vi "Experiment 26.vi"() -> ()   [LabVIEW 2026]
doc: "Experiment 26\nThis experiment (26) is like experiment 25 but uses 11 loops instead of 10. The subVIs in the first five loops use \"Same as caller\", and the last 6 loops use \"Other 1\"."
uses:
  <vilib>/AdvancedString/1D String Array to Delimited String (string).vi
  <vilib>/Analysis/baseanly.llb/Mean (DBL).vi
  <vilib>/Analysis/NI_AALBase.lvlib
panel:
  out "No. Of Iterations Executed - Loop 11":i32
  out "Output - Loop 11":dbl[](array[numeric]) format="%.3f"
  out "No. Of Iterations As Block Of Text (easy to copy into Excel)":string
  out "No. Of Iterations Executed - Loop 10":i32
  out "Output - Loop 10":dbl[](array[numeric]) format="%.3f"
  out "No. Of Iterations Executed - Loop 9":i32
  out "Output - Loop 9":dbl[](array[numeric]) format="%.3f"
  out "No. Of Iterations Executed - Loop 8":i32
  out "Output - Loop 8":dbl[](array[numeric]) format="%.3f"
  out "No. Of Iterations Executed - Loop 7":i32
  out "Output - Loop 7":dbl[](array[numeric]) format="%.3f"
  out "No. Of Iterations Executed - Loop 6":i32
  out "Output - Loop 6":dbl[](array[numeric]) format="%.3f"
  out "No. Of Iterations Executed - Loop 5":i32
  out "Output - Loop 5":dbl[](array[numeric]) format="%.3f"
  out "No. Of Iterations Executed - Loop 4":i32
  out "Output - Loop 4":dbl[](array[numeric]) format="%.3f"
  out "No. Of Iterations Executed - Loop 3":i32
  out "Output - Loop 3":dbl[](array[numeric]) format="%.3f"
  out "Avg. No. Of Iterations Executed - All Loops":dbl format="%.1f"
  out "No. Of Iterations Executed - Loop 2":i32
  out "Output - Loop 2":dbl[](array[numeric]) format="%.3f"
  out "No. Of Iterations Executed - Loop 1":i32
  out "Output - Loop 1":dbl[](array[numeric]) format="%.3f"
  out "Stop VI?":bool
  # "Experiment 26"
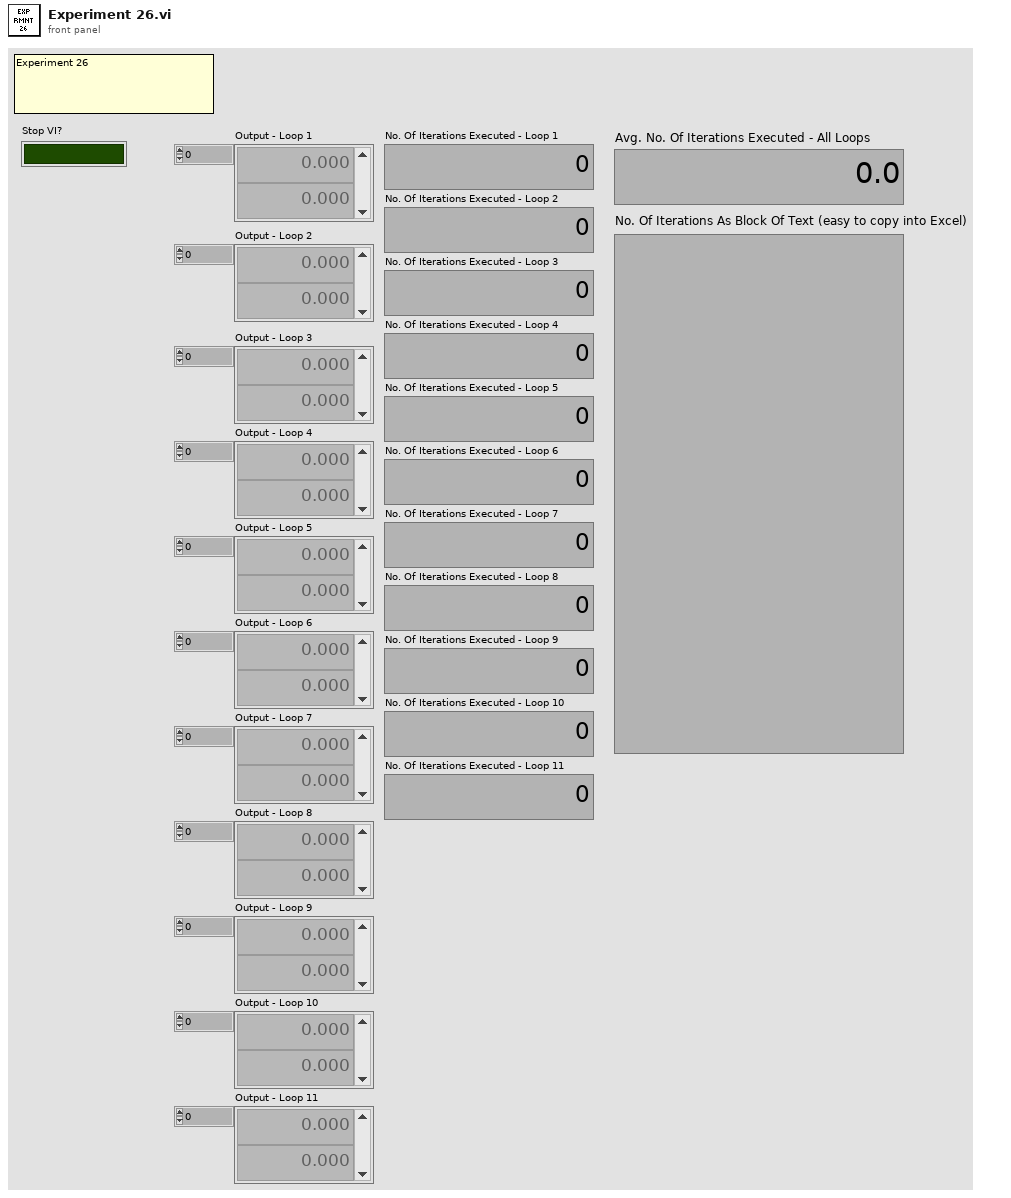
[diagram p1: front panel]
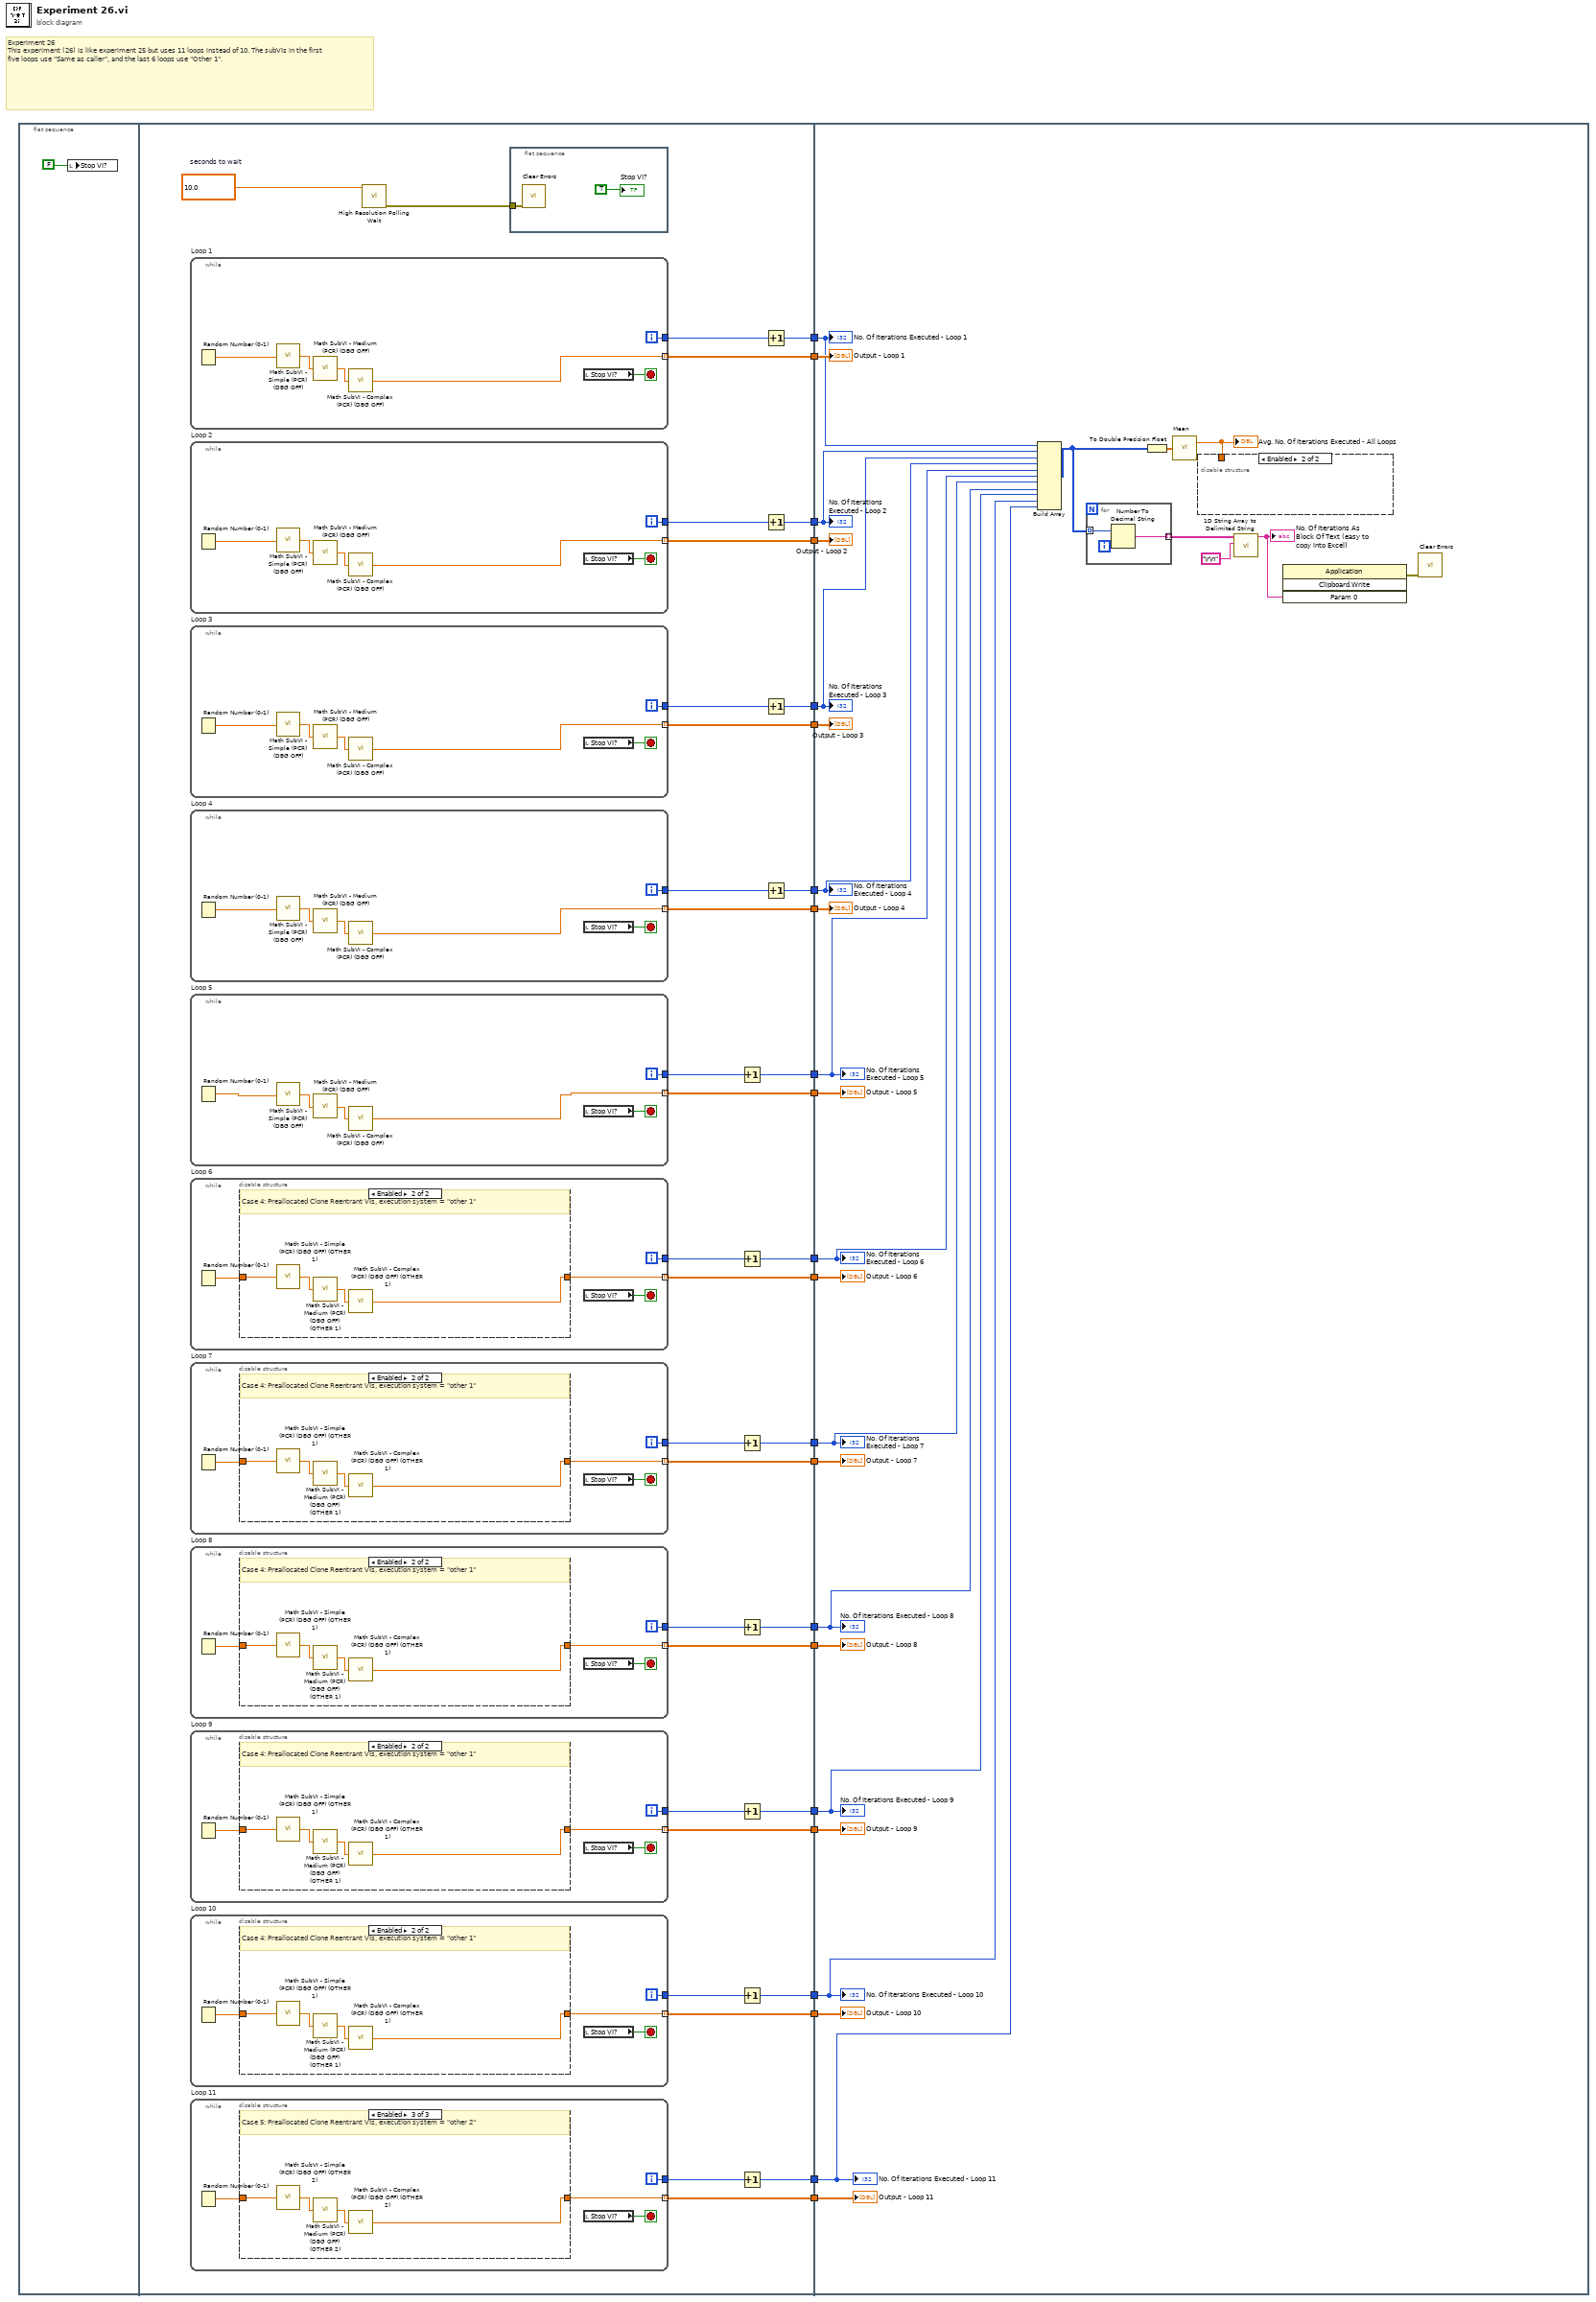
[diagram p0: block diagram]
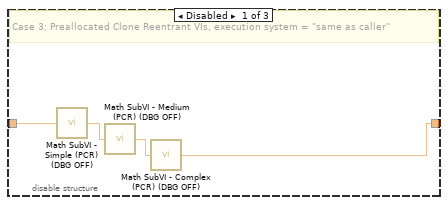
[diagram p2: hidden frame]
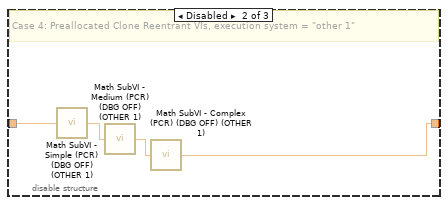
[diagram p3: hidden frame]
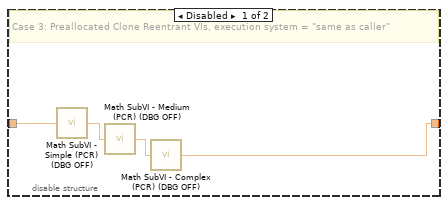
[diagram p4: hidden frame]
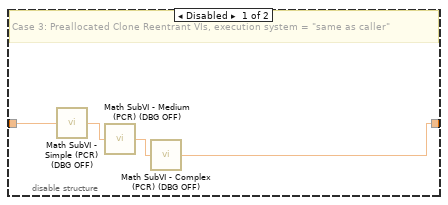
[diagram p5: hidden frame]
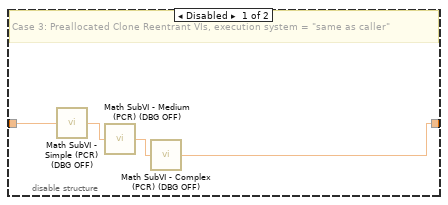
[diagram p6: hidden frame]
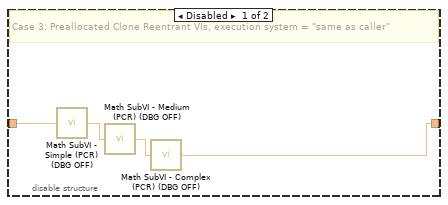
[diagram p7: hidden frame]
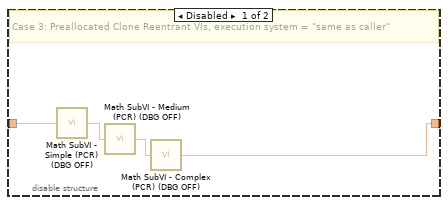
[diagram p8: hidden frame]
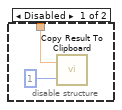
[diagram p9: hidden frame]
diagram:
  # "Experiment 26\nThis experiment (26) is like experiment 25 but uses 11 loops instead of 10. The subVIs in the first five loops use \"Same as caller\", and the last 6 loops use \"Other 1\"."
  n1 = flat-sequence {
    tunnel: [w56] -> w22
    tunnel: [w54] -> w21
    tunnel: [w53] -> w20
    tunnel: [w44] -> w19
    tunnel: [w52] -> w18
    tunnel: [w42] -> w17
    tunnel: [w40] -> w16
    tunnel: [w51] -> w15
    tunnel: [w38] -> w14
    tunnel: [w50] -> w13
    tunnel: [w36] -> w12
    tunnel: [w45] -> w11
    tunnel: [w34] -> w10
    tunnel: [w46] -> w9
    tunnel: [w32] -> w8
    tunnel: [w47] -> w7
    tunnel: [w30] -> w6
    tunnel: [w48] -> w5
    tunnel: [w27] -> w4
    tunnel: [w49] -> w3
    tunnel: [w26] -> w2
    tunnel: [w24] -> w1
    tunnel: w22 -> [w195]
    tunnel: w21 -> [w193]
    tunnel: w20 -> [w192]
    tunnel: w19 -> [w194]
    tunnel: w18 -> [w188]
    tunnel: w17 -> [w190]
    tunnel: w16 -> [w189]
    tunnel: w15 -> [w187]
    tunnel: w14 -> [w185]
    tunnel: w13 -> [w179]
    tunnel: w12 -> [w184]
    tunnel: w11 -> [w178]
    tunnel: w10 -> [w183]
    tunnel: w9 -> [w177]
    tunnel: w8 -> [w182]
    tunnel: w7 -> [w176]
    tunnel: w6 -> [w181]
    tunnel: w5 -> [w175]
    tunnel: w4 -> [w180]
    tunnel: w3 -> [w174]
    tunnel: w2 -> [w168]
    tunnel: w1 -> [w167]
    frame #0 {
      n2 = local write "Stop VI?"(FALSE) -> ()
    }
    frame #1 {
      w58 = 10.0  # seconds to wait
      n3 = while "Loop 1" {
        tunnel: [w162] -> w56 mode=indexing
        tunnel: [w163] -> w55
        i -> [w163]
        stop <- w164 stop-if-true
        n4 = Random Number (0-1)() -> (number: 0 to 1=w161:dbl)
        n5 = call "Math SubVI - Simple (PCR) (DBG OFF).vi"("Input"=w161) -> ("Output"=w159:dbl)
        n6 = call "Math SubVI - Medium (PCR) (DBG OFF).vi"("Input"=w159) -> ("Output"=w160:dbl)
        n7 = call "Math SubVI - Complex (PCR) (DBG OFF).vi"("Input"=w160) -> ("Output"=w162:dbl)
        n8 = local read "Stop VI?"() -> (w164:bool)
      }
      n9 = while "Loop 2" {
        tunnel: [w155] -> w44 mode=indexing
        tunnel: [w157] -> w43
        i -> [w157]
        stop <- w158 stop-if-true
        n10 = Random Number (0-1)() -> (number: 0 to 1=w156:dbl)
        n11 = call "Math SubVI - Simple (PCR) (DBG OFF).vi"("Input"=w156) -> ("Output"=w153:dbl)
        n12 = call "Math SubVI - Medium (PCR) (DBG OFF).vi"("Input"=w153) -> ("Output"=w154:dbl)
        n13 = call "Math SubVI - Complex (PCR) (DBG OFF).vi"("Input"=w154) -> ("Output"=w155:dbl)
        n14 = local read "Stop VI?"() -> (w158:bool)
      }
      n15 = while "Loop 3" {
        tunnel: [w149] -> w42 mode=indexing
        tunnel: [w151] -> w41
        i -> [w151]
        stop <- w152 stop-if-true
        n16 = Random Number (0-1)() -> (number: 0 to 1=w150:dbl)
        n17 = call "Math SubVI - Simple (PCR) (DBG OFF).vi"("Input"=w150) -> ("Output"=w147:dbl)
        n18 = call "Math SubVI - Medium (PCR) (DBG OFF).vi"("Input"=w147) -> ("Output"=w148:dbl)
        n19 = call "Math SubVI - Complex (PCR) (DBG OFF).vi"("Input"=w148) -> ("Output"=w149:dbl)
        n20 = local read "Stop VI?"() -> (w152:bool)
      }
      n21 = while "Loop 4" {
        tunnel: [w143] -> w40 mode=indexing
        tunnel: [w145] -> w39
        i -> [w145]
        stop <- w146 stop-if-true
        n22 = Random Number (0-1)() -> (number: 0 to 1=w144:dbl)
        n23 = call "Math SubVI - Simple (PCR) (DBG OFF).vi"("Input"=w144) -> ("Output"=w141:dbl)
        n24 = call "Math SubVI - Medium (PCR) (DBG OFF).vi"("Input"=w141) -> ("Output"=w142:dbl)
        n25 = call "Math SubVI - Complex (PCR) (DBG OFF).vi"("Input"=w142) -> ("Output"=w143:dbl)
        n26 = local read "Stop VI?"() -> (w146:bool)
      }
      n27 = while "Loop 5" {
        tunnel: [w137] -> w38 mode=indexing
        tunnel: [w139] -> w37
        i -> [w139]
        stop <- w140 stop-if-true
        n28 = Random Number (0-1)() -> (number: 0 to 1=w138:dbl)
        n29 = call "Math SubVI - Simple (PCR) (DBG OFF).vi"("Input"=w138) -> ("Output"=w135:dbl)
        n30 = call "Math SubVI - Medium (PCR) (DBG OFF).vi"("Input"=w135) -> ("Output"=w136:dbl)
        n31 = call "Math SubVI - Complex (PCR) (DBG OFF).vi"("Input"=w136) -> ("Output"=w137:dbl)
        n32 = local read "Stop VI?"() -> (w140:bool)
      }
      n33 = while "Loop 6" {
        tunnel: [w123] -> w36 mode=indexing
        tunnel: [w125] -> w35
        i -> [w125]
        stop <- w126 stop-if-true
        n34 = Random Number (0-1)() -> (number: 0 to 1=w124:dbl)
        n35 = disable-structure shown="Enabled" {
          disable-tunnel: w124 -> [w130 w134]
          disable-tunnel: [w129 w133] -> w123
          frame Disabled {
            # "Case 3: Preallocated Clone Reentrant VIs, execution system = \"same as caller\""
            n36 = call "Math SubVI - Simple (PCR) (DBG OFF).vi"("Input"=w130) -> ("Output"=w127:dbl)
            n37 = call "Math SubVI - Medium (PCR) (DBG OFF).vi"("Input"=w127) -> ("Output"=w128:dbl)
            n38 = call "Math SubVI - Complex (PCR) (DBG OFF).vi"("Input"=w128) -> ("Output"=w129:dbl)
          }
          frame Enabled {
            # "Case 4: Preallocated Clone Reentrant VIs, execution system = \"other 1\""
            n39 = call "Math SubVI - Simple (PCR) (DBG OFF) (OTHER 1).vi"("Input"=w134) -> ("Output"=w131:dbl)
            n40 = call "Math SubVI - Medium (PCR) (DBG OFF) (OTHER 1).vi"("Input"=w131) -> ("Output"=w132:dbl)
            n41 = call "Math SubVI - Complex (PCR) (DBG OFF) (OTHER 1).vi"("Input"=w132) -> ("Output"=w133:dbl)
          }
        }
        n42 = local read "Stop VI?"() -> (w126:bool)
      }
      n43 = while "Loop 7" {
        tunnel: [w111] -> w34 mode=indexing
        tunnel: [w113] -> w33
        i -> [w113]
        stop <- w114 stop-if-true
        n44 = Random Number (0-1)() -> (number: 0 to 1=w112:dbl)
        n45 = disable-structure shown="Enabled" {
          disable-tunnel: w112 -> [w118 w122]
          disable-tunnel: [w117 w121] -> w111
          frame Disabled {
            # "Case 3: Preallocated Clone Reentrant VIs, execution system = \"same as caller\""
            n46 = call "Math SubVI - Simple (PCR) (DBG OFF).vi"("Input"=w118) -> ("Output"=w115:dbl)
            n47 = call "Math SubVI - Medium (PCR) (DBG OFF).vi"("Input"=w115) -> ("Output"=w116:dbl)
            n48 = call "Math SubVI - Complex (PCR) (DBG OFF).vi"("Input"=w116) -> ("Output"=w117:dbl)
          }
          frame Enabled {
            # "Case 4: Preallocated Clone Reentrant VIs, execution system = \"other 1\""
            n49 = call "Math SubVI - Simple (PCR) (DBG OFF) (OTHER 1).vi"("Input"=w122) -> ("Output"=w119:dbl)
            n50 = call "Math SubVI - Medium (PCR) (DBG OFF) (OTHER 1).vi"("Input"=w119) -> ("Output"=w120:dbl)
            n51 = call "Math SubVI - Complex (PCR) (DBG OFF) (OTHER 1).vi"("Input"=w120) -> ("Output"=w121:dbl)
          }
        }
        n52 = local read "Stop VI?"() -> (w114:bool)
      }
      n53 = while "Loop 8" {
        tunnel: [w99] -> w32 mode=indexing
        tunnel: [w101] -> w31
        i -> [w101]
        stop <- w102 stop-if-true
        n54 = Random Number (0-1)() -> (number: 0 to 1=w100:dbl)
        n55 = disable-structure shown="Enabled" {
          disable-tunnel: w100 -> [w106 w110]
          disable-tunnel: [w105 w109] -> w99
          frame Disabled {
            # "Case 3: Preallocated Clone Reentrant VIs, execution system = \"same as caller\""
            n56 = call "Math SubVI - Simple (PCR) (DBG OFF).vi"("Input"=w106) -> ("Output"=w103:dbl)
            n57 = call "Math SubVI - Medium (PCR) (DBG OFF).vi"("Input"=w103) -> ("Output"=w104:dbl)
            n58 = call "Math SubVI - Complex (PCR) (DBG OFF).vi"("Input"=w104) -> ("Output"=w105:dbl)
          }
          frame Enabled {
            # "Case 4: Preallocated Clone Reentrant VIs, execution system = \"other 1\""
            n59 = call "Math SubVI - Simple (PCR) (DBG OFF) (OTHER 1).vi"("Input"=w110) -> ("Output"=w107:dbl)
            n60 = call "Math SubVI - Medium (PCR) (DBG OFF) (OTHER 1).vi"("Input"=w107) -> ("Output"=w108:dbl)
            n61 = call "Math SubVI - Complex (PCR) (DBG OFF) (OTHER 1).vi"("Input"=w108) -> ("Output"=w109:dbl)
          }
        }
        n62 = local read "Stop VI?"() -> (w102:bool)
      }
      n63 = while "Loop 9" {
        tunnel: [w87] -> w30 mode=indexing
        tunnel: [w89] -> w29
        i -> [w89]
        stop <- w90 stop-if-true
        n64 = Random Number (0-1)() -> (number: 0 to 1=w88:dbl)
        n65 = disable-structure shown="Enabled" {
          disable-tunnel: w88 -> [w94 w98]
          disable-tunnel: [w93 w97] -> w87
          frame Disabled {
            # "Case 3: Preallocated Clone Reentrant VIs, execution system = \"same as caller\""
            n66 = call "Math SubVI - Simple (PCR) (DBG OFF).vi"("Input"=w94) -> ("Output"=w91:dbl)
            n67 = call "Math SubVI - Medium (PCR) (DBG OFF).vi"("Input"=w91) -> ("Output"=w92:dbl)
            n68 = call "Math SubVI - Complex (PCR) (DBG OFF).vi"("Input"=w92) -> ("Output"=w93:dbl)
          }
          frame Enabled {
            # "Case 4: Preallocated Clone Reentrant VIs, execution system = \"other 1\""
            n69 = call "Math SubVI - Simple (PCR) (DBG OFF) (OTHER 1).vi"("Input"=w98) -> ("Output"=w95:dbl)
            n70 = call "Math SubVI - Medium (PCR) (DBG OFF) (OTHER 1).vi"("Input"=w95) -> ("Output"=w96:dbl)
            n71 = call "Math SubVI - Complex (PCR) (DBG OFF) (OTHER 1).vi"("Input"=w96) -> ("Output"=w97:dbl)
          }
        }
        n72 = local read "Stop VI?"() -> (w90:bool)
      }
      n73 = while "Loop 10" {
        tunnel: [w75] -> w27 mode=indexing
        tunnel: [w77] -> w28
        i -> [w77]
        stop <- w78 stop-if-true
        n74 = Random Number (0-1)() -> (number: 0 to 1=w76:dbl)
        n75 = disable-structure shown="Enabled" {
          disable-tunnel: w76 -> [w82 w86]
          disable-tunnel: [w81 w85] -> w75
          frame Disabled {
            # "Case 3: Preallocated Clone Reentrant VIs, execution system = \"same as caller\""
            n76 = call "Math SubVI - Simple (PCR) (DBG OFF).vi"("Input"=w82) -> ("Output"=w79:dbl)
            n77 = call "Math SubVI - Medium (PCR) (DBG OFF).vi"("Input"=w79) -> ("Output"=w80:dbl)
            n78 = call "Math SubVI - Complex (PCR) (DBG OFF).vi"("Input"=w80) -> ("Output"=w81:dbl)
          }
          frame Enabled {
            # "Case 4: Preallocated Clone Reentrant VIs, execution system = \"other 1\""
            n79 = call "Math SubVI - Simple (PCR) (DBG OFF) (OTHER 1).vi"("Input"=w86) -> ("Output"=w83:dbl)
            n80 = call "Math SubVI - Medium (PCR) (DBG OFF) (OTHER 1).vi"("Input"=w83) -> ("Output"=w84:dbl)
            n81 = call "Math SubVI - Complex (PCR) (DBG OFF) (OTHER 1).vi"("Input"=w84) -> ("Output"=w85:dbl)
          }
        }
        n82 = local read "Stop VI?"() -> (w78:bool)
      }
      n83 = while "Loop 11" {
        tunnel: [w59] -> w26 mode=indexing
        tunnel: [w61] -> w25
        i -> [w61]
        stop <- w62 stop-if-true
        n84 = Random Number (0-1)() -> (number: 0 to 1=w60:dbl)
        n85 = disable-structure shown="Enabled" {
          disable-tunnel: w60 -> [w66 w70 w74]
          disable-tunnel: [w65 w69 w73] -> w59
          frame Disabled {
            # "Case 3: Preallocated Clone Reentrant VIs, execution system = \"same as caller\""
            n86 = call "Math SubVI - Simple (PCR) (DBG OFF).vi"("Input"=w66) -> ("Output"=w63:dbl)
            n87 = call "Math SubVI - Medium (PCR) (DBG OFF).vi"("Input"=w63) -> ("Output"=w64:dbl)
            n88 = call "Math SubVI - Complex (PCR) (DBG OFF).vi"("Input"=w64) -> ("Output"=w65:dbl)
          }
          frame Disabled {
            # "Case 4: Preallocated Clone Reentrant VIs, execution system = \"other 1\""
            n89 = call "Math SubVI - Simple (PCR) (DBG OFF) (OTHER 1).vi"("Input"=w70) -> ("Output"=w67:dbl)
            n90 = call "Math SubVI - Medium (PCR) (DBG OFF) (OTHER 1).vi"("Input"=w67) -> ("Output"=w68:dbl)
            n91 = call "Math SubVI - Complex (PCR) (DBG OFF) (OTHER 1).vi"("Input"=w68) -> ("Output"=w69:dbl)
          }
          frame Enabled {
            # "Case 5: Preallocated Clone Reentrant VIs, execution system = \"other 2\""
            n92 = call "Math SubVI - Simple (PCR) (DBG OFF) (OTHER 2).vi"("Input"=w74) -> ("Output"=w71:dbl)
            n93 = call "Math SubVI - Medium (PCR) (DBG OFF) (OTHER 2).vi"("Input"=w71) -> ("Output"=w72:dbl)
            n94 = call "Math SubVI - Complex (PCR) (DBG OFF) (OTHER 2).vi"("Input"=w72) -> ("Output"=w73:dbl)
          }
        }
        n95 = local read "Stop VI?"() -> (w62:bool)
      }
      n96 = call <vilib>:"High Resolution Polling Wait.vi"("seconds to wait"=w58) -> ("error out"=w57:errorcluster)  [unwired: 10 in]
      n97 = flat-sequence {
        tunnel: w57 -> [w165]
        frame #0 {
          n98 = call <vilib>:"Clear Errors.vi"("error in (no error)"=w165) -> ()  [unwired: 5 in, 2 out]
          "Stop VI?" <- TRUE
        }
      }
      n99 = Increment(x=w37) -> (x+1=w50:i32)
      n100 = Increment(x=w35) -> (x+1=w45:i32)
      n101 = Increment(x=w33) -> (x+1=w46:i32)
      n102 = Increment(x=w31) -> (x+1=w47:i32)
      n103 = Increment(x=w29) -> (x+1=w48:i32)
      n104 = Increment(x=w28) -> (x+1=w49:i32)
      n105 = Increment(x=w25) -> (x+1=w24:i32)
      n106 = Increment(x=w55) -> (x+1=w54:i32)
      n107 = Increment(x=w43) -> (x+1=w53:i32)
      n108 = Increment(x=w41) -> (x+1=w52:i32)
      n109 = Increment(x=w39) -> (x+1=w51:i32)
    }
    frame #2 {
      n110 = Build Array(w193, w192, w188, w187, w179, w178, w177, w176, w175, w174, w167) -> (w173:i32[])
      n111 = for {
        tunnel: w173 -> [w199] mode=indexing
        tunnel: [w198] -> w172 mode=indexing
        n112 = Number To Decimal String(number=w199) -> (decimal integer string=w198:string)  [unwired: 1 in]
      }
      n113 = To Double Precision Float(number=w173) -> (double precision float=w186:dbl[])
      n114 = call-poly <vilib>:"Mean.vi"("X"=w186) -> ("mean"=w191:dbl)  [unwired: 1 out]
      "Avg. No. Of Iterations Executed - All Loops" <- w191
      n115 = disable-structure shown="Enabled" {
        disable-tunnel: w191 -> [w197 _]
        frame Disabled {
          n116 = call "Copy Result To Clipboard.vi"("No. Of Decimal Places (6)"=u32 1, "Input"=w197) -> ()
        }
        frame Enabled {
        }
      }
      n117 = call-poly <vilib>:"1D String Array to Delimited String.vi"("delimiter"="\r\n", "string array"=w172) -> ("delimited string"=w169:string)  [unwired: 9 in]
      "No. Of Iterations As Block Of Text (easy to copy into Excel)" <- w169
      n118 = invoke class="Application" method="Clipboard.Write"("Param 0"=w169) -> (error out=w170:errorcluster)  [unwired: 3 in, 3 out]
      n119 = call <vilib>:"Clear Errors.vi"("error in (no error)"=w170) -> ()  [unwired: 5 in, 2 out]
      "No. Of Iterations Executed - Loop 1" <- w193
      "Output - Loop 1" <- w195
      "No. Of Iterations Executed - Loop 2" <- w192
      "Output - Loop 2" <- w194
      "No. Of Iterations Executed - Loop 3" <- w188
      "Output - Loop 3" <- w190
      "No. Of Iterations Executed - Loop 4" <- w187
      "Output - Loop 4" <- w189
      "No. Of Iterations Executed - Loop 5" <- w179
      "Output - Loop 5" <- w185
      "No. Of Iterations Executed - Loop 6" <- w178
      "Output - Loop 6" <- w184
      "No. Of Iterations Executed - Loop 7" <- w177
      "Output - Loop 7" <- w183
      "No. Of Iterations Executed - Loop 8" <- w176
      "Output - Loop 8" <- w182
      "No. Of Iterations Executed - Loop 9" <- w175
      "Output - Loop 9" <- w181
      "No. Of Iterations Executed - Loop 10" <- w174
      "Output - Loop 10" <- w180
      "No. Of Iterations Executed - Loop 11" <- w167
      "Output - Loop 11" <- w168
    }
  }
